vi "CUSTOM_CHIP.vi"(0 "Camera Handle":u32, 1 "Window Size":u32, 2 "TriggerMode":u32, 4 "Vertical Clock":u32, 5 "error out":errorcluster, 6 "Pre Y":u32, 7 "Pre X":u32, 8 "Enable / Disable Custom Chip":bool=TRUE, 9 "ReadOut Mode":u16(ring)=1 items=["Full Frame"=1, "Kinetics"=10], 10 "Post Y":u32, 11 "Post X":u32, 12 "Parallel (Y) Size":u32, 13 "Serial (X) Size":u32) -> (14 "Camera Handle":u32, 15 "INI Flag":bool, 18 "String":string, 19 "error out":errorcluster)   [LabVIEW 2015]
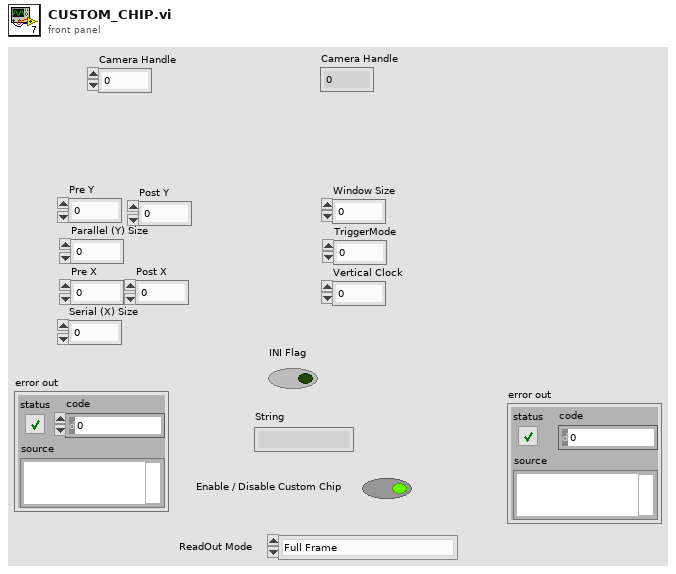
[diagram p1: front panel]
types:
  T1 = cluster{"Pre Y":u32, "Post Y":u32, "Parallel (Y) Size":u32, "Pre X":u32, "Post X":u32, "Serial (X) Size":u32}
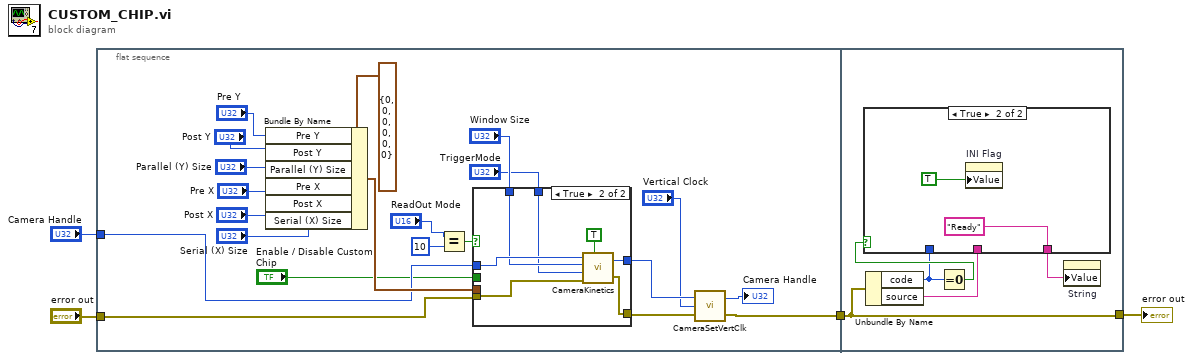
[diagram p0: block diagram]
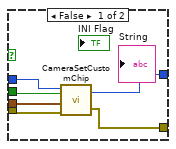
[diagram p2: hidden frame]
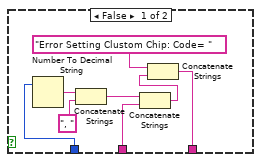
[diagram p3: hidden frame]
diagram:
  n1 = flat-sequence {
    tunnel: [w25] -> w4
    tunnel: "error out" -> [w22]
    tunnel: "Camera Handle" -> [w17]
    tunnel: w4 -> [w43]
    tunnel: [w43] -> w2
    frame #0 {
      n2 = Bundle By Name(cluster=T1 {"Pre Y"=0, "Post Y"=0, "Parallel (Y) Size"=0, "Pre X"=0, "Post X"=0, "Serial (X) Size"=0} ("Custom Chip Settings"), "Pre Y"="Pre Y", "Post Y"="Post Y", "Parallel (Y) Size"="Parallel (Y) Size", "Pre X"="Pre X", "Post X"="Post X", "Serial (X) Size"="Serial (X) Size") -> (w19:T1)
      n3 = Equal?(x="ReadOut Mode", y=10) -> (x = y?=w24:bool)
      n4 = case shown="True" w24 {
        tunnel: w22 -> [w31 w38]
        tunnel: [w30 w37] -> w21
        tunnel: w19 -> [w29 _]
        tunnel: "Enable / Disable Custom Chip" -> [w28 _]
        tunnel: [w27 w35] -> w18
        tunnel: w17 -> [w26 w34]
        tunnel: "Window Size" -> [_ w33]
        tunnel: "TriggerMode" -> [_ w32]
        frame False {
          n5 = call <userlib>:"CameraSetCustomChip.vi"("error in (no error)"=w31, "Custom Chip Settings"=w29, "Enable/Disable Custom Chip"=w28, "Camera Handle"=w26) -> ("error out"=w30:errorcluster, "Camera Handle"=w27:u32)
        }
        frame True {
          n6 = call <userlib>:"CameraKinetics.vi"("Camera Handle"=w34, "Window Size"=w33, "TriggerMode"=w32, "error in (no error)"=w38, "Enable/Disable Kinetics"=TRUE) -> ("Camera Handle"=w35:u32, "error out"=w37:errorcluster)
        }
      }
      n7 = call <userlib>:"CameraSetVertClk.vi"("error in (no error)"=w21, "Vertical Clock"="Vertical Clock", "Camera Handle"=w18) -> ("error out"=w25:errorcluster, "Camera Handle"=→"Camera Handle":u32)
    }
    frame #1 {
      n8 = Unbundle By Name(w43) -> ("code"=w40:i32, "source"=w41:string)
      n9 = Equal To 0?(x=w40) -> (x = 0?=w42:bool)
      n10 = case shown="True" w42 {
        tunnel: [w44 "Ready"] -> w39
        tunnel: w41 -> [w45 _]
        tunnel: w40 -> [w50 _]
        frame False {
          n11 = Number To Decimal String(number=w50) -> (decimal integer string=w49:string)  [unwired: 1 in]
          n12 = Concatenate Strings(w49, ", ") -> (w46:string)
          n13 = Concatenate Strings(w46, w45) -> (w47:string)
          n14 = Concatenate Strings("Error Setting Clustom Chip: Code= ", w47) -> (w44:string)
        }
        frame True {
          n15 = property on="INI Flag" class="Bool (strict)"("Value"=TRUE) -> ()  [unwired: 2 in, 2 out]
        }
      }
      n16 = property on="String" class="Str"("Value"=w39) -> ()  [unwired: 2 in, 2 out]
    }
  }
  "error out" <- w2
